vi "FB Switch Input Const No Var.vi"(8 "error in":errorcluster) -> (0 "error out":errorcluster, 3 "data out":variant)   [LabVIEW 2020]
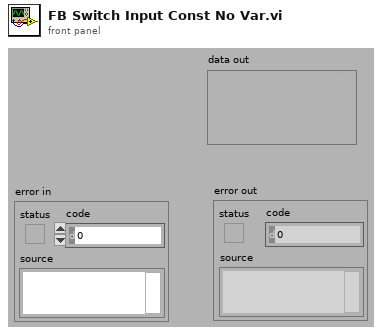
[diagram p1: front panel]
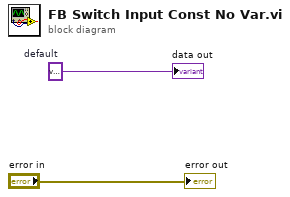
[diagram p0: block diagram]
diagram:
  w1 = variant  # default
  "data out" <- w1
  "error out" <- "error in"
